vi "Get Windows.vi"(8 "error in (no error)":errorcluster, 11 "Head Impulse Fit in":refnum<class "Head Impulse Fit.lvclass">) -> (0 "error out":errorcluster, 1 "Window Length":i32, 2 "Window Start Indicies":i32[](array[numeric]), 3 "Head Impulse Fit out":refnum<class "Head Impulse Fit.lvclass">)   [LabVIEW 2016, in "Head Impulse Fit.lvclass"]
uses:
  Head Impulse Fit.lvclass
  Head Impulse Fit.lvclass/Head Impulse Fit.ctl
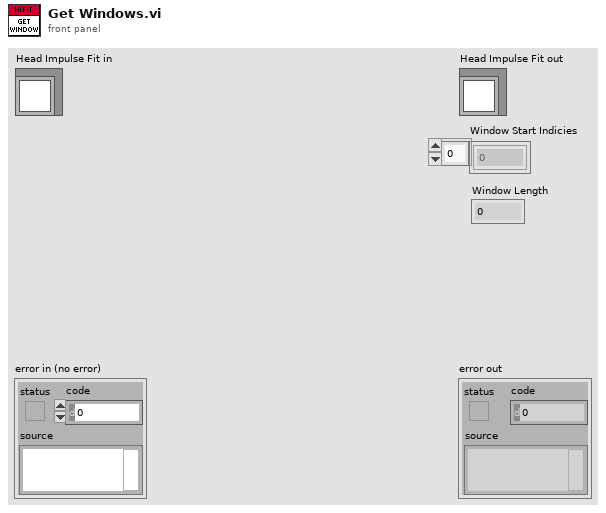
[diagram p1: front panel]
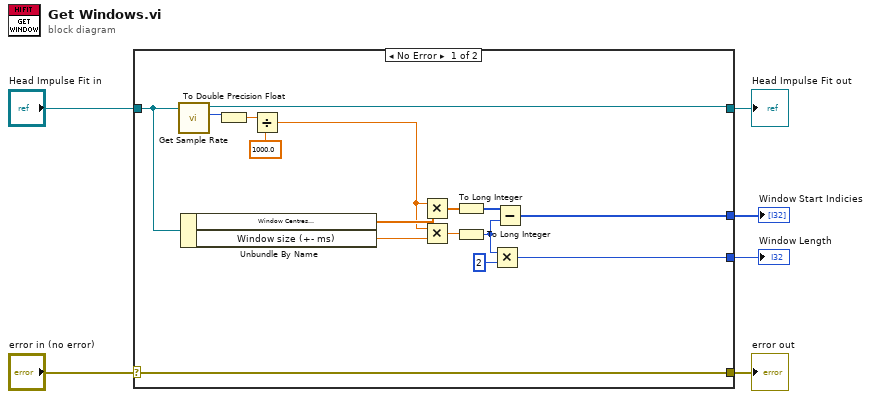
[diagram p0: block diagram]
diagram:
  n1 = case shown="No Error" "error in (no error)" {
    selector: "error in (no error)" -> [w22 w24]
    tunnel: [w22 w24] -> w5
    tunnel: [w8 w23] -> w3
    tunnel: "Head Impulse Fit in" -> [w18 w23]
    tunnel: [w9 _] -> w2
    tunnel: [w7 _] -> w1
    frame No Error {
      n2 = call-dynamic "Get Sample Rate.vi"("Abstract Fit in"=w18) -> ("Sample Rate"=w19:i32, "Abstract Fit out"=w8:refnum<class "Head Impulse Fit.lvclass">)  [unwired: 8 in, 1 out]
      n3 = Unbundle By Name(w18) -> ("Window Centres\n(ms after onset)"=w12:dbl[], "Window size (+- ms)"=w11:dbl)
      n4 = To Double Precision Float(number=w19) -> (double precision float=w21:dbl)
      n5 = Divide(x=w21, y=1000.0) -> (x/y=w10:dbl)
      n6 = Multiply(x=w10, y=w12) -> (x*y=w14:dbl[])
      n7 = Multiply(x=w10, y=w11) -> (x*y=w13:dbl)
      n8 = To Long Integer(number=w14) -> (32bit integer=w16:i32[])
      n9 = To Long Integer(number=w13) -> (32bit integer=w17:i32)
      n10 = Multiply(x=w17, y=2) -> (x*y=w7:i32)
      n11 = Subtract(x=w16, y=w17) -> (x-y=w9:i32[])
    }
    frame Error {
    }
  }
  "error out" <- w5
  "Head Impulse Fit out" <- w3
  "Window Start Indicies" <- w2
  "Window Length" <- w1
